vi "setShiftSpeed.vi"(8 "error in (no error)":errorcluster, 10 "Shift Speed":T1={"Vertical Shift Speed"=0.525, "Horizontal Shift Speed"=2.5, "Fast Kinetic V Shift Speed"=0.0}, 11 "CameraSettingsManager.lvclass in":refnum<class "CameraSettingsManager.lvclass">) -> (0 "error out":errorcluster, 3 "CameraSettingsManager.lvclass out":refnum<class "CameraSettingsManager.lvclass">)   [LabVIEW 2009, in "Tools.lvlib" / "Settings.lvlib" / "CameraSettingsManager.lvclass"]
uses:
  CameraSettingsManager.lvclass
  CameraSettingsManager.lvclass/CameraSettingsManager.ctl
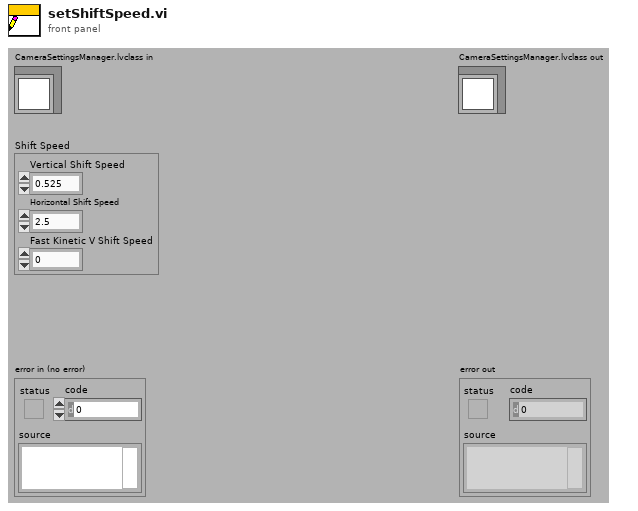
[diagram p1: front panel]
types:
  T1 = cluster{"Vertical Shift Speed":dbl, "Horizontal Shift Speed":dbl, "Fast Kinetic V Shift Speed":dbl}
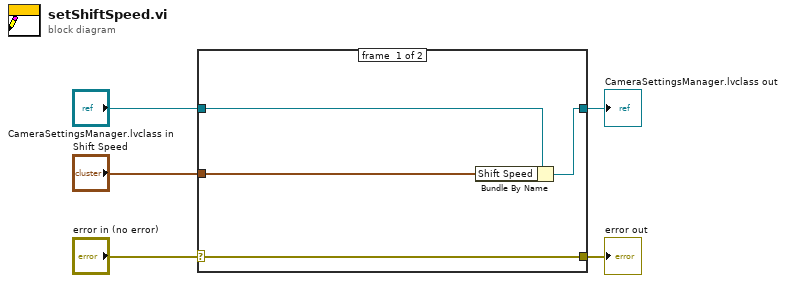
[diagram p0: block diagram]
diagram:
  n1 = case shown="No Error" "error in (no error)" {
    selector: "error in (no error)" -> [w9 w10]
    tunnel: [w9 w10] -> w4
    tunnel: [w7 w11] -> w2
    tunnel: "CameraSettingsManager.lvclass in" -> [w8 w11]
    tunnel: "Shift Speed" -> [w6 _]
    frame #0 {
      n2 = Bundle By Name(cluster=w8, "Shift Speed"=w6) -> (w7:refnum<class "CameraSettingsManager.lvclass">)
    }
    frame #1 {
    }
  }
  "error out" <- w4
  "CameraSettingsManager.lvclass out" <- w2
